vi "WriteDB.vi"() -> ()   [LabVIEW 2018]
uses:
  <vilib>/addons/database/Connection.llb/DB Tools Open Connec (Path).vi
  <vilib>/addons/database/NI_Database_API.lvlib
panel:
  in  "Columns":string[](array[string])=["cMacCode", "cInvCode", "cCheckDate", "cCheckNo", "cState", "cDefine1", "cDefine2", "cDefine3", "cDefine4", "cDefine5", "cDefine6", "cDefine7", "cDefine8", "cDefine9", "cDefine10", "cDefine11", "cDefine12", "cDefine13", "cDefine14", "cDefine15", "cDefine16", "cDefine17", "cDefine18"]
  in  "SQL_Data":T1={"cMacCode"="1-C-225", "cInvCode"="820901", "cCheckDate"="2018-10-29 16:05:31", "cCheckNo"="2018102900005", "cState"="OK", "cDefine1"="OK", "cDefine2"="OK", "cDefine3"="OK", "cDefine4"="OK", "cDefine5"="OK", "cDefine6"="OK", "cDefine7"="", "cDefine8"="OK", "cDefine9"=2.56, "cDefine10"=2.43, "cDefine11"=4.05, "cDefine12"=0.56, "cDefine13"=1.0, "cDefine14"=1.0, "cDefine15"="OK", "cDefine16"="OK", "cDefine17"="OK", "cDefine18"="OK"}
  out "error out":errorcluster
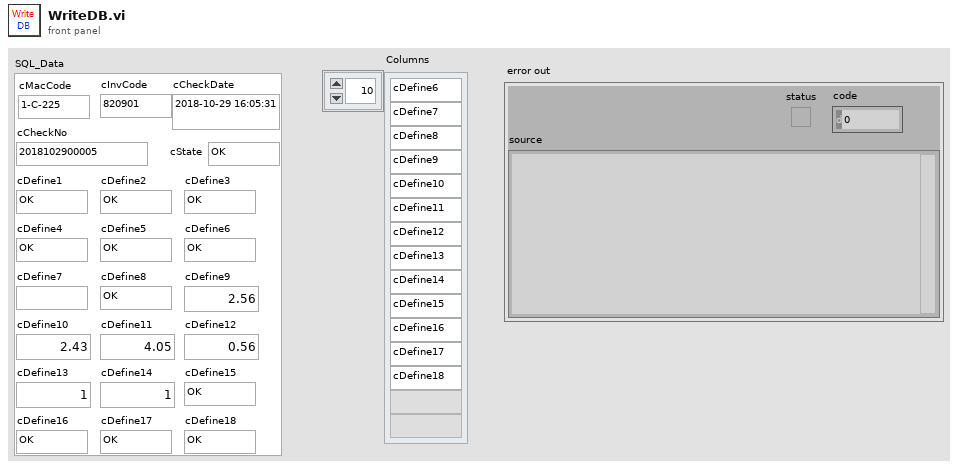
[diagram p1: front panel]
types:
  T1 = cluster{"cMacCode":string, "cInvCode":string, "cCheckDate":string, "cCheckNo":string, "cState":string, "cDefine1":string, "cDefine2":string, "cDefine3":string, "cDefine4":string, "cDefine5":string, "cDefine6":string, "cDefine7":string, "cDefine8":string, "cDefine9":dbl, "cDefine10":dbl, "cDefine11":dbl, "cDefine12":dbl, "cDefine13":dbl, "cDefine14":dbl, "cDefine15":string, "cDefine16":string, "cDefine17":string, "cDefine18":string}
  T2 = typedef "NI_Database_API.lvlib/Conn ObjectReference.ctl" = refnum<k1>
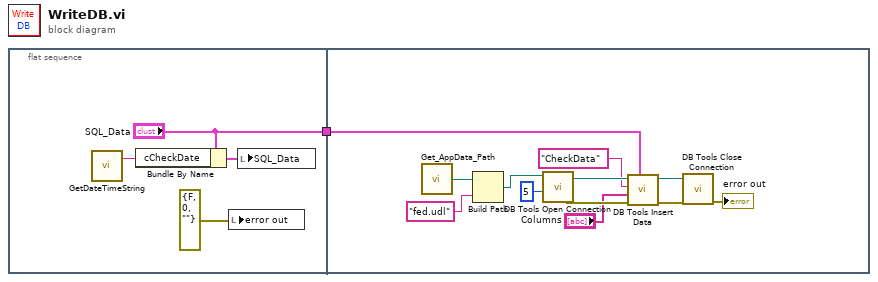
[diagram p0: block diagram]
diagram:
  n1 = flat-sequence {
    tunnel: ["SQL_Data"] -> w1
    tunnel: w1 -> [w6]
    frame #0 {
      n2 = call "GetDateTimeString.vi"() -> ("date/time string"=w2:string)  [unwired: 4 in, 1 out]
      n3 = Bundle By Name(cluster="SQL_Data", "cCheckDate"=w2) -> (w5:T1)
      n4 = local write "error out"(errorcluster {"status"=FALSE, "code"=0, "source"=""} ("错误常量")) -> ()
      n5 = local write "SQL_Data"(w5) -> ()
    }
    frame #1 {
      n6 = call "Get_AppData_Path.vi"() -> ("path"=w16:path)  [unwired: 1 in]
      n7 = Build Path(base path=w16, name or relative path="fed.udl" ("名称或相对路径")) -> (appended path=w15:path)
      n8 = call-poly <vilib>:"DB Tools Open Connection.vi"("connection timeout (15)"=5, "connection information"=w15) -> ("error out"=w10:errorcluster, "connection reference"=w12:T2)  [unwired: 6 in]
      n9 = call <vilib>:"DB Tools Insert Data.vi"("data"=w6, "error in (no error)"=w10, "columns"="Columns", "table"="CheckData", "connection reference"=w12) -> ("error out"=w9:errorcluster, "connection reference out"=w11:T2)  [unwired: 5 in]
      n10 = call <vilib>:"DB Tools Close Connection.vi"("error in (no error)"=w9, "connection reference"=w11) -> ("error out"=→"error out":errorcluster)  [unwired: 5 in]
    }
  }
